vi "Save Config.vi"(8 "error in (no error)":errorcluster, 10 "FileName":string="SerialConfig.xml", 11 "DeviceList":T1[](array[typedef])) -> (0 "error out":errorcluster)   [LabVIEW 2010, in "MonitorServer.lvlib"]
doc: "Use this template to build a VI to use as a subVI."
uses:
  MonitorServer.lvlib
  Serial Config.ctl
  <vilib>/Utility/xml.llb/Write to XML File(string).vi
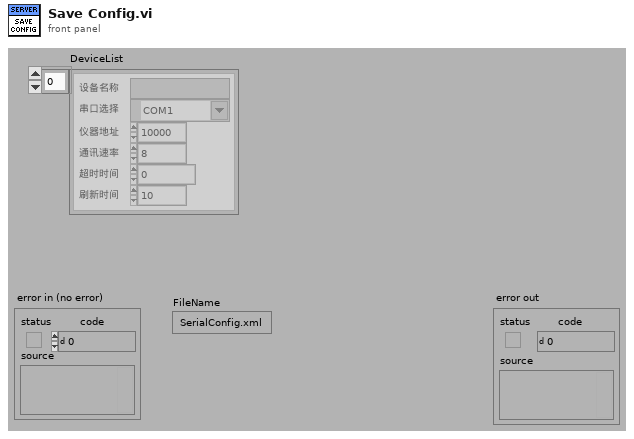
[diagram p1: front panel]
types:
  T1 = typedef "MonitorServer.lvlib/Serial Config.ctl" = cluster{"设备名称":string, "串口选择":refnum<visa-resource-name>, "仪器地址":u32, "通讯速率":u32, "超时时间":u32, "刷新时间":dbl}
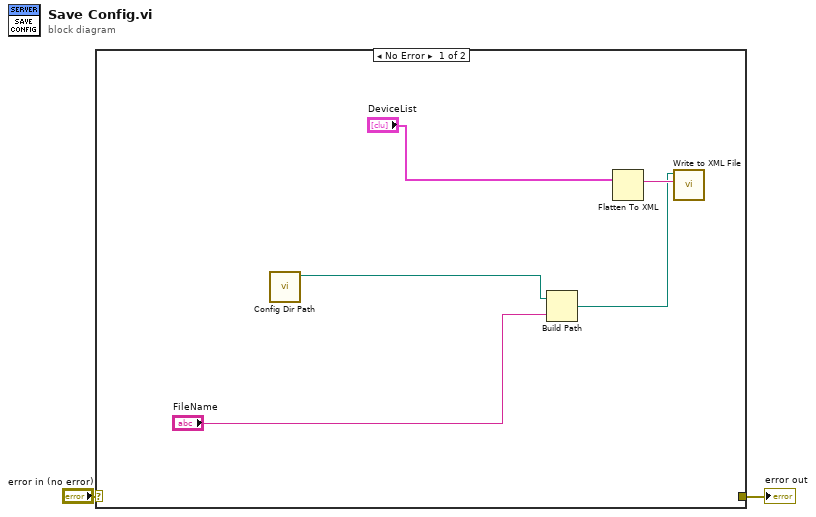
[diagram p0: block diagram]
diagram:
  n1 = case shown="No Error" "error in (no error)" {
    selector: "error in (no error)" -> [_ w8]
    tunnel: [_ w8] -> w1
    frame No Error {
      n2 = call "Config Dir Path.vi"() -> ("App.Dir"=w6:path)  [unwired: 11 in]
      n3 = Build Path(base path=w6, name or relative path="FileName") -> (appended path=w4:path)
      n4 = Flatten To XML(anything="DeviceList") -> (xml string=w7:string)
      n5 = call-poly <vilib>:"Write to XML File.vi"("XML Input"=w7, "XML File Path"=w4) -> ()  [unwired: 7 in, 3 out]
    }
    frame Error {
    }
  }
  "error out" <- w1
